vi "Coil Dynamic Event FGV.vi"(7 "Action":enum16{"Create", "Get", "Destroy"}(ring)=enum."Destroy", 8 "error in (no error)":errorcluster) -> (0 "error out":errorcluster, 2 "coil event":refnum<user-event>)   [LabVIEW 2021]
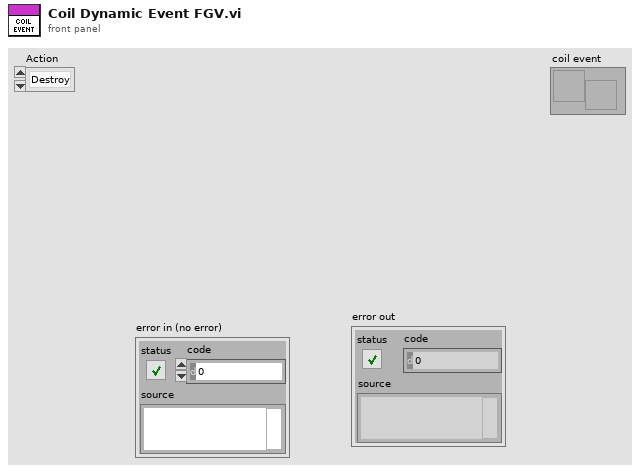
[diagram p1: front panel]
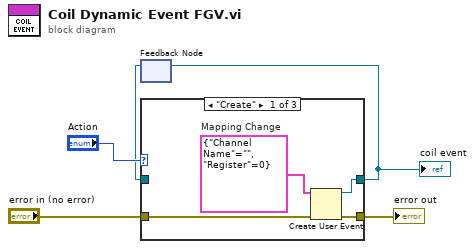
[diagram p0: block diagram]
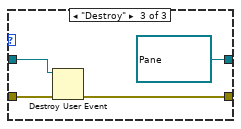
[diagram p3: hidden frame]
diagram:
  n1 = feedback #1() -> (w3:refnum<user-event>)  [unwired: 1 in]
  n2 = case shown="\"Create\"" "Action" {
    tunnel: [w8 w11 refnum<user-event> refnum ("user event")] -> w4
    tunnel: w3 -> [_ w11 w15]
    tunnel: "error in (no error)" -> [w7 w10 w13]
    tunnel: [w6 w10 w12] -> w1
    frame "Create" {
      w9 = cluster{"Channel Name":string, "Register":u16} {"Channel Name"="", "Register"=0}  # Mapping Change
      n3 = Create User Event(user event datatype=w9, error in=w7) -> (user event=w8:refnum<user-event>, error out=w6:errorcluster)
    }
    frame "Get" {
    }
    frame "Destroy" {
      n4 = Destroy User Event(user event=w15, error in=w13) -> (error out=w12:errorcluster)
    }
  }
  "error out" <- w1
  "coil event" <- w4
  n5 = feedback-in #1(w4) -> ()
